vi "Normalize Coordinates with Angle.vi"(8 "navX Attitude":T1, 9 "Camera Type":T2, 10 "Targets":T5(array[cluster]), 11 "Image in":T6) -> (0 "Camera Position Y":dbl, 1 "Camera Position X":dbl, 2 "Found Targets":T3(array[cluster]) {"Normalized Rect"."Lower Border" format="%#_2g"; "Normalized Rect"."Right Border" format="%#_2g"; "Normalized Rect"."Top Border" format="%#_2g"; "Normalized Rect"."Left Border" format="%#_2g"}, 3 "Sorted Scores":T4(array[cluster]) {"Moment Factor" format="%#_3g"; "L" format="%#_3g"; "Area to CH" format="%#_3g"; "X" format="%#_3g"; "Y" format="%#_3g"}, 4 "Angle to Target":dbl)   [LabVIEW 2023]
doc: "Normalize the rectangle and center so that they range from -1 to 1, left to right and bottom to top. This helps with producing joystick coordinates for driving the robot and makes the code better at handling resolution changes of the camera."
uses:
  <vilib>/vision/Image Controls.llb/IMAQ Image.ctl
  Camera Types.ctl
  D:/2017/Software Stuff/1094 Robot Code/Robot-Dashboard Shared Files/navX Attitude.ctl
panel:
  # "Aspect Ratio"
  # "Density Profile"
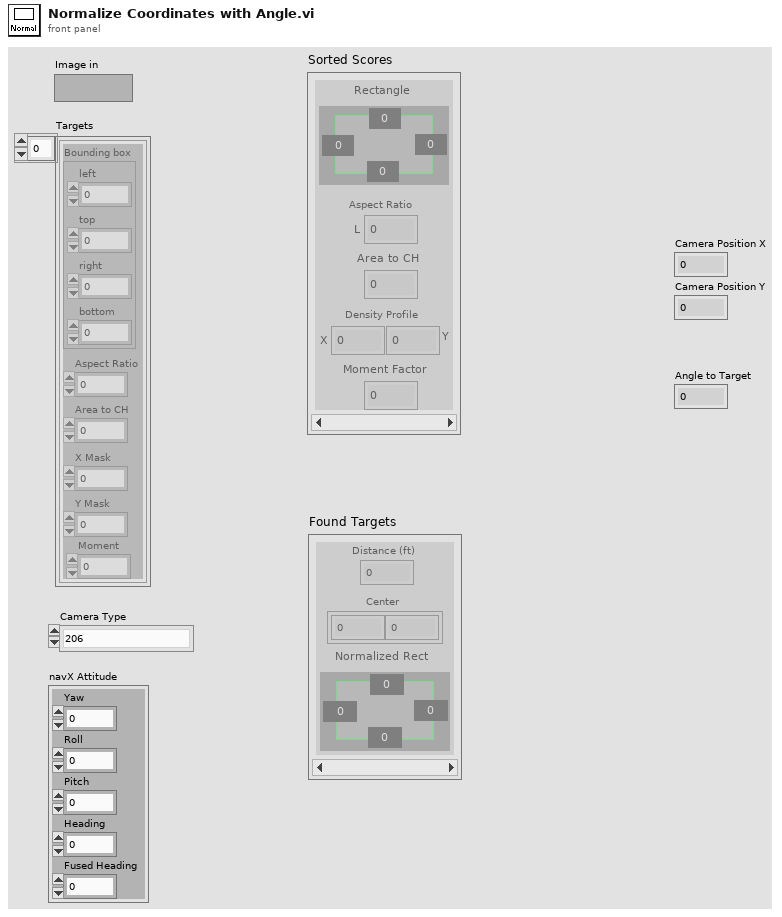
[diagram p1: front panel]
types:
  T1 = typedef "navX Attitude.ctl" = cluster{"Yaw":dbl, "Roll":dbl, "Pitch":dbl, "Heading":dbl, "Fused Heading":dbl}
  T2 = typedef "Camera Types.ctl" = enum16{"206", "1011", "1013", "MS HD3000 square", "MS HD3000 640x480", "MS HD3000 1280x720"}
  T3 = cluster{"Distance (ft)":dbl, "Center":cluster{dbl, dbl}, "Normalized Rect":cluster{"Left Border":dbl, "Top Border":dbl, "Right Border":dbl, "Lower Border":dbl}}[]
  T4 = cluster{"Rectangle":cluster{"Numeric":dbl, "Numeric 2":dbl, "Numeric 3":dbl, "Numeric 5":dbl}, "L":dbl, "Area to CH":dbl, "X":dbl, "Y":dbl, "Moment Factor":dbl}[]
  T5 = cluster{"Bounding box":cluster{"left":dbl, "top":dbl, "right":dbl, "bottom":dbl}, "Aspect Ratio":dbl, "Area to CH":dbl, "X Mask":dbl, "Y Mask":dbl, "Moment":dbl}[]
  T6 = typedef "IMAQ Image.ctl" = refnum<image>
  T7 = cluster{"Left":dbl, "Top":dbl, "Right":dbl, "Bottom":dbl}
  T8 = cluster{"left":dbl, "top":dbl, "right":dbl, "bottom":dbl}
  T9 = cluster{"X Resolution":i32, i32, "X Resolution":i32, i32}
  T10 = cluster{"Image Dst Out":T6, cluster{dbl, dbl}, cluster{dbl, dbl, dbl, dbl}}
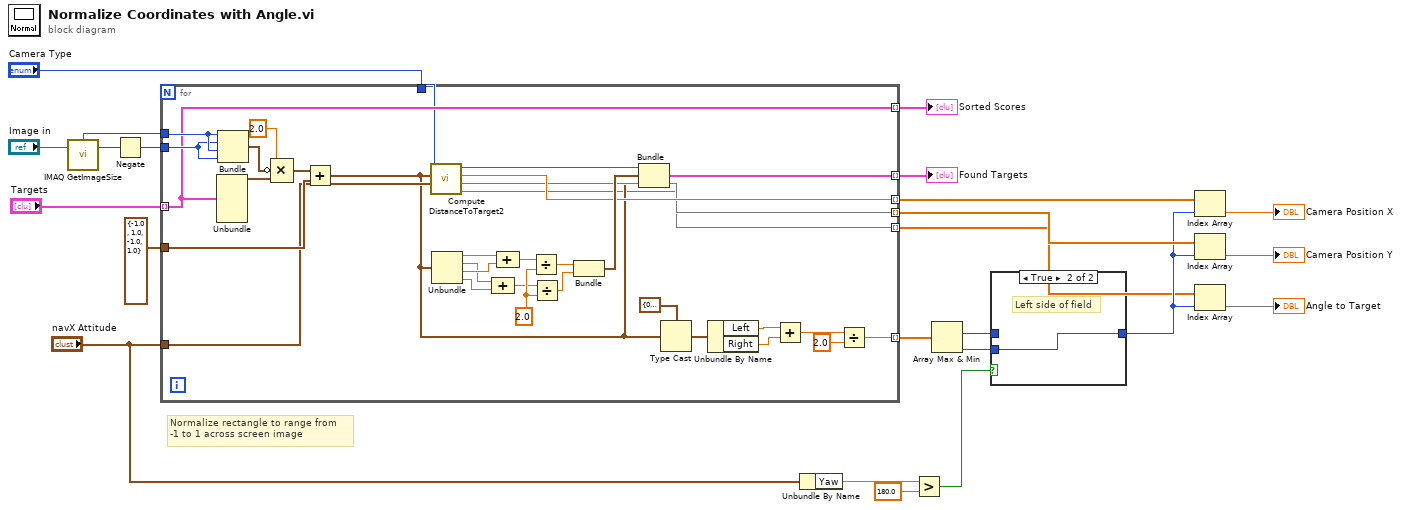
[diagram p0: block diagram]
diagram:
  # "Normalize rectangle to range from\n-1 to 1 across screen image"
  n1 = call "IMAQ GetImageSize"("Image"="Image in") -> ("Y Resolution"=w21:i32, "X Resolution"=w22:i32)  [unwired: 3 in, 1 out]
  n2 = Negate(x=w21) -> (-x=w23:i32)
  n3 = for {
    tunnel: "Targets" -> [w38] mode=indexing
    tunnel: w23 -> [w55]
    tunnel: w22 -> [w56]
    tunnel: [w41] -> w10 mode=indexing
    tunnel: [w38] -> w11 mode=indexing
    tunnel: cluster{dbl, dbl, dbl, dbl} {-1.0, 1.0, -1.0, 1.0} ("y") -> [w37]
    tunnel: "Camera Type" -> [w36]
    tunnel: [w35] -> w15 mode=indexing
    tunnel: [w34] -> w14 mode=indexing
    tunnel: "navX Attitude" -> [w33]
    tunnel: [w25] -> w5 mode=indexing
    tunnel: [w24] -> w2 mode=indexing
    w46 = 2.0
    n4 = Unbundle(w38) -> ("Bounding box"=w53:T8)  [unwired: 5 out]
    n5 = Bundle("X Resolution"=w56, w55, "X Resolution"=w56, w55) -> (w54:T9)  [unwired: 1 in]
    n6 = Compound Arithmetic op=MULTIPLY(2.0, invert w54, w53) -> (w52:cluster{dbl, dbl, dbl, dbl})
    n7 = Add(x=w52, y=w37) -> (x+y=w31:cluster{dbl, dbl, dbl, dbl})
    n8 = call "Compute DistanceToTarget2.vi"("Camera Type"=w33, "Line"=w31, "Image Src"=w36) -> (0:w24, 1:w34, "Distance (ft)"=w35:dbl, "Image Dst Out"=w40:T6)  [unwired: 5 in]
    n9 = Unbundle(w31) -> (w50:dbl, w47:dbl, w49:dbl, w48:dbl)
    n10 = Compound Arithmetic op=ADD(w47, w48) -> (w44:dbl)
    n11 = Compound Arithmetic op=ADD(w50, w49) -> (w45:dbl)
    n12 = Divide(x=w45, y=w46) -> (x/y=w43:dbl)
    n13 = Divide(x=w44, y=w46) -> (x/y=w42:dbl)
    n14 = Bundle(w43, w42) -> (w39:cluster{dbl, dbl})  [unwired: 1 in]
    n15 = Bundle("Image Dst Out"=w40, w39, w31) -> (w41:T10)  [unwired: 1 in]
    n16 = Type Cast(type=T7 {"Left"=0.0, "Top"=0.0, "Right"=0.0, "Bottom"=0.0} ("Normalized Rect"), x=w31) -> (*(type *) &x=w30:T7)
    n17 = Unbundle By Name(w30) -> ("Left"=w29:dbl, "Right"=w28:dbl)
    n18 = Add(x=w29, y=w28) -> (x+y=w27:dbl)
    n19 = Divide(x=w27, y=2.0) -> (x/y=w25:dbl)
  }
  "Sorted Scores" <- w11
  "Found Targets" <- w10
  n20 = Unbundle By Name("navX Attitude") -> ("Yaw"=w3:dbl)
  n21 = Greater?(x=w3, y=180.0) -> (0:w6:bool)
  n22 = Array Max & Min(array=w5) -> (max index (indices)=w8:i32, min index (indices)=w7:i32)  [unwired: 2 out]
  n23 = case shown="True" w6 {
    tunnel: w8 -> [w57 _]
    tunnel: w7 -> [_ w58]
    tunnel: [w57 w58] -> w4
    frame False {
      # "Right side of field"
    }
    frame True {
      # "Left side of field"
    }
  }
  n24 = Index Array(array=w15, index=w4) -> (element=→"Camera Position X":dbl)
  n25 = Index Array(array=w14, index=w4) -> (element=→"Camera Position Y")
  n26 = Index Array(array=w2, index=w4) -> (element=→"Angle to Target")
